vi "Check Register Request.vi"(9 "Sequence":u32, 10 "Send Message Data":T1, 11 "Request Queue":refnum<queue>) -> (1 "Seq dup":u32)   [LabVIEW 2020, in "Vecto.lvlib" / "TCPMessaging.lvclass"]
uses:
  TCPMessaging.lvclass
  lv-promises/Promises/Promise/Promise.lvclass
  Request Registration.ctl
  proto/TcpPayload/Data.ctl
  proto/TcpPayload/TcpPayload.lvlib
  Send Message Data.ctl
  Vecto.lvlib
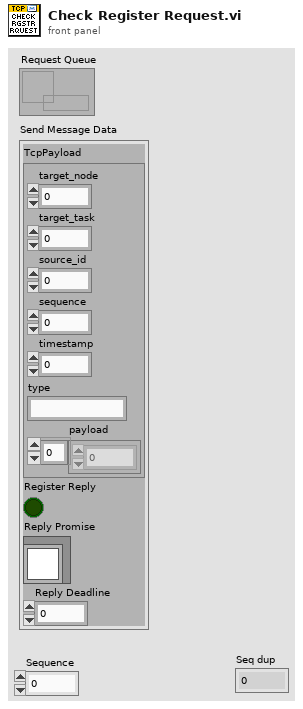
[diagram p1: front panel]
types:
  T1 = typedef "Vecto.lvlib/Send Message Data.ctl" = cluster{"TcpPayload":T2, "Register Reply":bool, "Reply Promise":refnum<class "Promise.lvclass">, "Reply Deadline":dbl}
  T2 = typedef "TcpPayload.lvlib/Data.ctl" = cluster{"target_node":u32, "target_task":u32, "source_id":u32, "sequence":u32, "timestamp":u64, "type":string, "payload":u8[]}
  T3 = typedef "Vecto.lvlib/TCPMessaging.lvclass/Request Registration.ctl" = cluster{"Sequence":u32, "Reply Promise":refnum<class "Promise.lvclass">, "Reply Deadline":dbl}
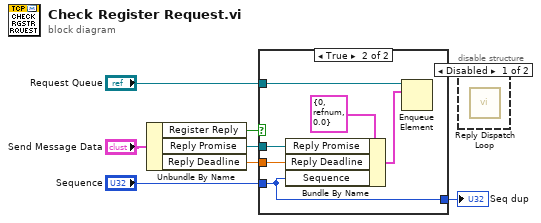
[diagram p0: block diagram]
diagram:
  n1 = Unbundle By Name("Send Message Data") -> ("Register Reply"=w7:bool, "Reply Promise"=w6:refnum<class "Promise.lvclass">, "Reply Deadline"=w5:dbl)
  n2 = case shown="True" w7 {
    tunnel: "Sequence" -> [w8 w9]
    tunnel: w5 -> [_ w13]
    tunnel: w6 -> [_ w14]
    tunnel: "Request Queue" -> [_ w12]
    tunnel: [w8 w9] -> w1
    frame False {
    }
    frame True {
      n3 = Bundle By Name(cluster=T3 {"Sequence"=0, "Reply Promise"=refnum, "Reply Deadline"=0.0} ("Request Registration"), "Reply Promise"=w14, "Reply Deadline"=w13, "Sequence"=w9) -> (w10:T3)
      n4 = Enqueue Element(queue=w12, element=w10) -> ()  [unwired: 2 in, 3 out]
    }
  }
  "Seq dup" <- w1
  n5 = disable-structure shown="Disabled" {
    frame Disabled {
      n6 = call "Reply Dispatch Loop.vi"() -> ()  [unwired: 11 in, 1 out]
    }
    frame Enabled {
    }
  }
